vi "PAN_inspectName.vi"(4 "cmdline name":string, 6 "pan config dir":path, 8 "error in (no error)":errorcluster, 10 "name in":string) -> (0 "error out":errorcluster, 2 "name out":string)   [LabVIEW 2016]
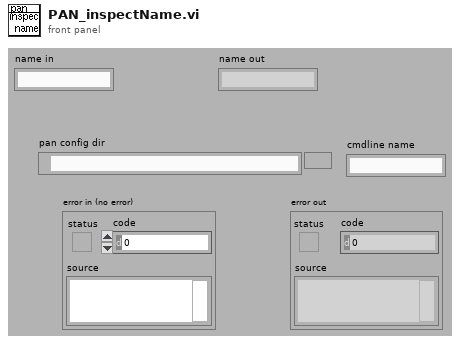
[diagram p1: front panel]
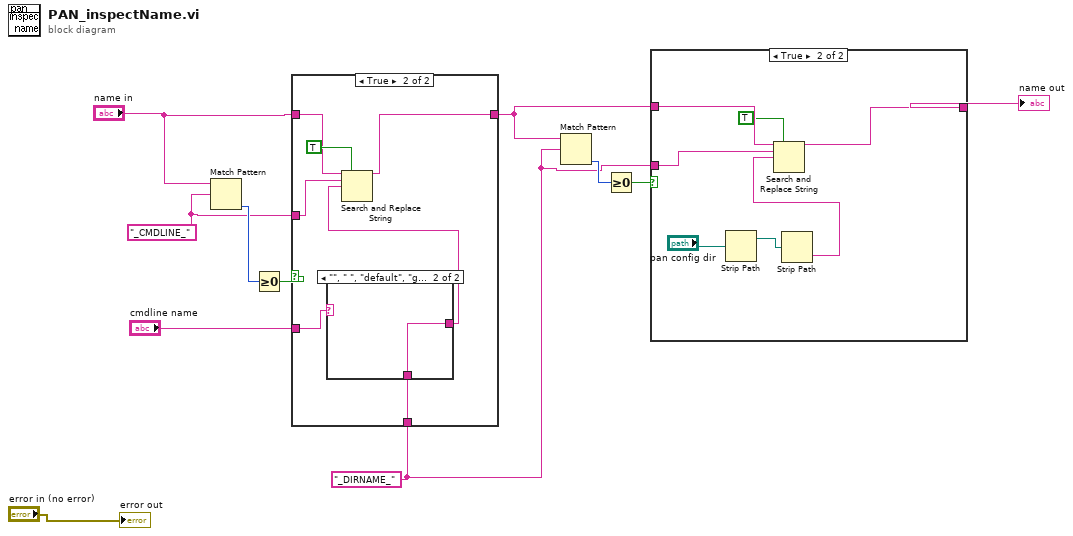
[diagram p0: block diagram]
diagram:
  w2 = "_DIRNAME_" ("regular expression")
  w3 = "_CMDLINE_" ("regular expression")
  n1 = Match Pattern(string="name in", regular expression=w3) -> (offset past match=w8:i32)  [unwired: 4 out]
  n2 = Greater Or Equal To 0?(x=w8) -> (x >= 0?=w7:bool)
  n3 = case shown="True" w7 {
    tunnel: "name in" -> [w12 w18]
    tunnel: [w12 w16] -> w5
    tunnel: "cmdline name" -> [_ w15]
    tunnel: w3 -> [_ w17]
    tunnel: w2 -> [_ w13]
    frame False {
    }
    frame True {
      n4 = case shown="\"\", \" \", \"default\", \"generic\"" w15 {
        selector: w15 -> [w20 _]
        tunnel: [w20 w21] -> w14
        tunnel: w13 -> [_ w21]
        frame Default {
        }
        frame "", " ", "default", "generic" {
        }
      }
      n5 = Search and Replace String(replace all?=TRUE ("replace all? (F)"), input string=w18, search string=w17, replace string=w14) -> (result string=w16:string)  [unwired: 1 in, 6 out]
    }
  }
  n6 = Match Pattern(string=w5, regular expression=w2) -> (offset past match=w11:i32)  [unwired: 4 out]
  n7 = Greater Or Equal To 0?(x=w11) -> (x >= 0?=w10:bool)
  n8 = case shown="True" w10 {
    tunnel: [w22 w24] -> w9
    tunnel: w5 -> [w22 w27]
    tunnel: w2 -> [_ w26]
    frame False {
    }
    frame True {
      n9 = Strip Path(path="pan config dir") -> (stripped path=w28:path)  [unwired: 1 out]
      n10 = Strip Path(path=w28) -> (name=w25:string)  [unwired: 1 out]
      n11 = Search and Replace String(replace all?=TRUE ("replace all? (F)"), input string=w27, search string=w26, replace string=w25) -> (result string=w24:string)  [unwired: 1 in, 6 out]
    }
  }
  "name out" <- w9
  "error out" <- "error in (no error)"
